vi "MQTT_PUBLISH.vi"(6 "MSG":string, 7 "Enviar":bool, 8 "error in (no error)":errorcluster, 9 "TOPIC":string, 10 "IP":string, 11 "VISA resource name":refnum<visa-resource-name>) -> (0 "error out":errorcluster, 3 "VISA resource name out":refnum<visa-resource-name>)   [LabVIEW 2025]
panel:
  out "read buffer":string
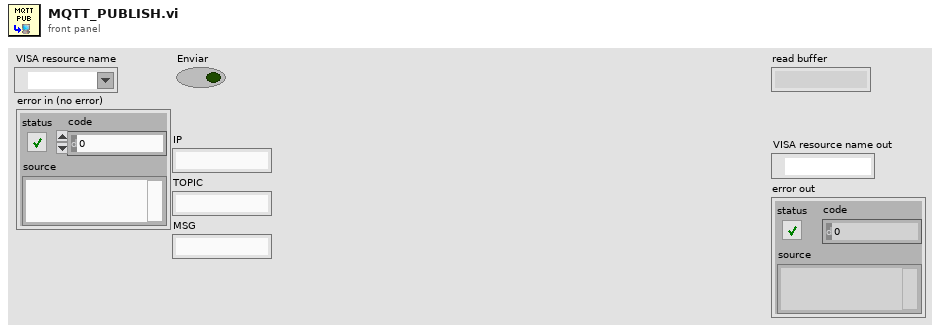
[diagram p1: front panel]
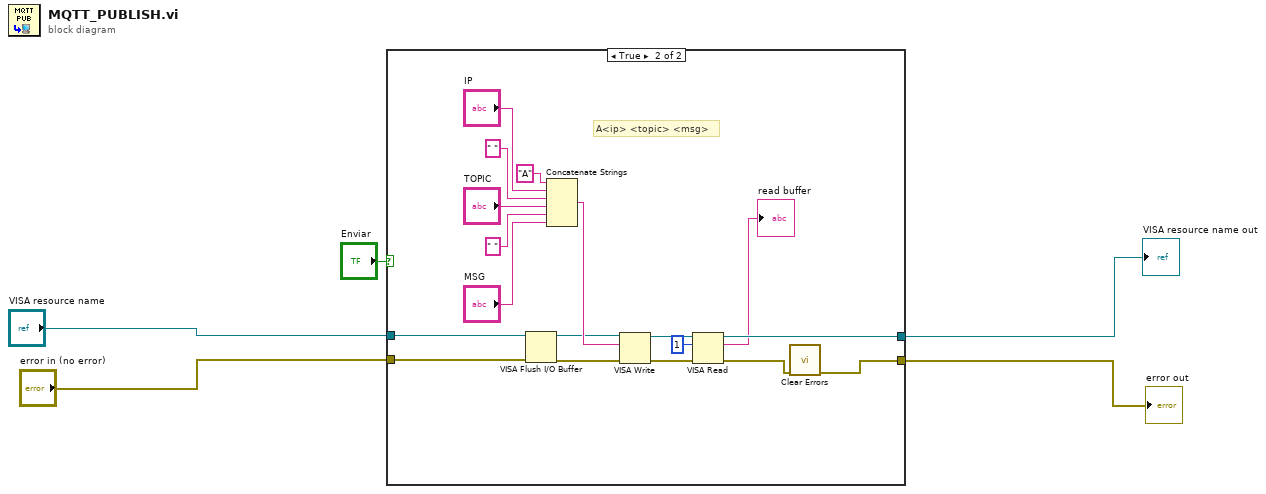
[diagram p0: block diagram]
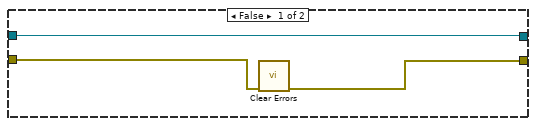
[diagram p2: hidden frame]
diagram:
  n1 = case shown="True" "Enviar" {
    tunnel: [w8 w16] -> w5
    tunnel: [w7 w10] -> w4
    tunnel: "error in (no error)" -> [w6 w13]
    tunnel: "VISA resource name" -> [w8 w12]
    frame False {
      n2 = call <vilib>:"Clear Errors.vi"("error in (no error)"=w6) -> ("error out"=w7:errorcluster)  [unwired: 5 in, 1 out]
    }
    frame True {
      # "A<ip> <topic> <msg>"
      n3 = VISA Flush I/O Buffer(VISA resource name=w12, error in (no error)=w13) -> (VISA resource name out=w15:refnum<visa-resource-name>, error out=w14:errorcluster)  [unwired: 1 in]
      n4 = Concatenate Strings("A", "IP", " " ("string"), "TOPIC", " " ("string"), "MSG") -> (w21:string)
      n5 = VISA Write(VISA resource name=w15, write buffer=w21, error in (no error)=w14) -> (VISA resource name out=w25:refnum<visa-resource-name>, error out=w26:errorcluster)  [unwired: 1 out]
      n6 = VISA Read(VISA resource name=w25, byte count=u32 1, error in (no error)=w26) -> (VISA resource name out=w16:refnum<visa-resource-name>, read buffer=→"read buffer":string, error out=w9:errorcluster)  [unwired: 1 out]
      n7 = call <vilib>:"Clear Errors.vi"("error in (no error)"=w9) -> ("error out"=w10:errorcluster)  [unwired: 5 in, 1 out]
    }
  }
  "VISA resource name out" <- w5
  "error out" <- w4
